vi "Hello World.vi"() -> ()   [LabVIEW 2017]
panel:
  out "String 2":string
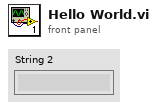
[diagram p1: front panel]
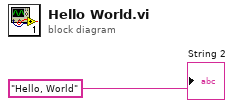
[diagram p0: block diagram]
diagram:
  "String 2" <- "Hello, World"
